vi "Tape on off.vi"(7 "Settings":T1={"max velocity"={"Value"=0.0, "Min"=0.0, "Max"=0.0, "StepSize"=0.0, "Tolerance"=0.0, "ValueActual"=0.0}, "continious velocity"={"Value"=0.0, "Min"=0.0, "Max"=0.0, "StepSize"=0.0, "Tolerance"=0.0, "ValueActual"=0.0}, "shake"=enum."off", "direction"=enum."left", "RedRatio"={"Value"=0.0, "Min"=0.0, "Max"=0.0, "StepSize"=0.0, "Tolerance"=0.0, "ValueActual"=0.0}, "StepSize"={"Value"=0.0, "Min"=0.0, "Max"=0.0, "StepSize"=0.0, "Tolerance"=0.0, "ValueActual"=0.0}, "position"={"Value"=0.0, "Min"=0.0, "Max"=0.0, "StepSize"=0.0, "Tolerance"=0.0, "ValueActual"=0.0}, "velocity"={"Value"=0.0, "Min"=0.0, "Max"=0.0, "StepSize"=0.0, "Tolerance"=0.0, "ValueActual"=0.0}, "Step"=enum."off", "Mode"=enum."on demand", "timeout"={"Value"=0.0, "Min"=0.0, "Max"=0.0, "StepSize"=0.0, "Tolerance"=0.0, "ValueActual"=0.0}, "DelayStage"={"Value"=0.0, "Min"=0.0, "Max"=0.0, "StepSize"=0.0, "Tolerance"=0.0, "ValueActual"=0.0}, "TapeMotor"=enum."off", "encoder Axis"=0, "oldpos"=0.0, "ResetEncoder"=enum."off", "tape monitor"=enum."off", "ComPort"="", "Stream Settings"={"My Name"="", "Remote IP Address"="", "Remote Name"=""}, "Motor1Axis"=0, "Motor2Axis"=0, "OptimizeTensionAfterStep"=enum."off", "StepVelocity"={"Value"=0.0, "Min"=0.0, "Max"=0.0, "StepSize"=0.0, "Tolerance"=0.0, "ValueActual"=0.0}, "MotorDirection"=enum."left", "MinTapeMonMax"={"Value"=0.0, "Min"=0.0, "Max"=0.0, "StepSize"=0.0, "Tolerance"=0.0, "ValueActual"=0.0}, "NumberSubSteps"={"Value"=0.0, "Min"=0.0, "Max"=0.0, "StepSize"=0.0, "Tolerance"=0.0, "ValueActual"=0.0}, "SimpleMinTapeMonMaxCheck"=enum."off", "WaitBeforeScanStep"={"Value"=0.0, "Min"=0.0, "Max"=0.0, "StepSize"=0.0, "Tolerance"=0.0, "ValueActual"=0.0}, "MaxStepTries"={"Value"=100.0, "Min"=0.0, "Max"=0.0, "StepSize"=0.0, "Tolerance"=0.0, "ValueActual"=0.0}}, 8 "error in (no error)":errorcluster, 9 "Arg":string, 10 "String":string, 11 "VISA Refnum in":refnum<visa-resource-name>) -> (0 "error out":errorcluster, 2 "Velocity (units/s)":dbl, 3 "new commands":string)   [LabVIEW 2020, in "TapeDrive.lvclass"]
uses:
  TapeDrive.lvclass
  settings_TypDef.ctl
  shared/numericVariable_TypeDef.ctl
  shared/OnOffTypeDef.ctl
  Direction_TypDef.ctl
  Mode_TypDEf.ctl
  <vilib>/addons/_JKI.lib/Network_Streams_Connection.llb/PublicSettings.ctl
  shared/CompressAndUpdate(Poly)/CompressAndUpdate(Enum).vi
  Newport ESP301/Newport ESP301.lvlib
  BaseDriver/BaseDriver.lvclass
  <vilib>/addons/_JKI.lib/Network_Streams_Connection.llb/NetworkConnection.lvclass
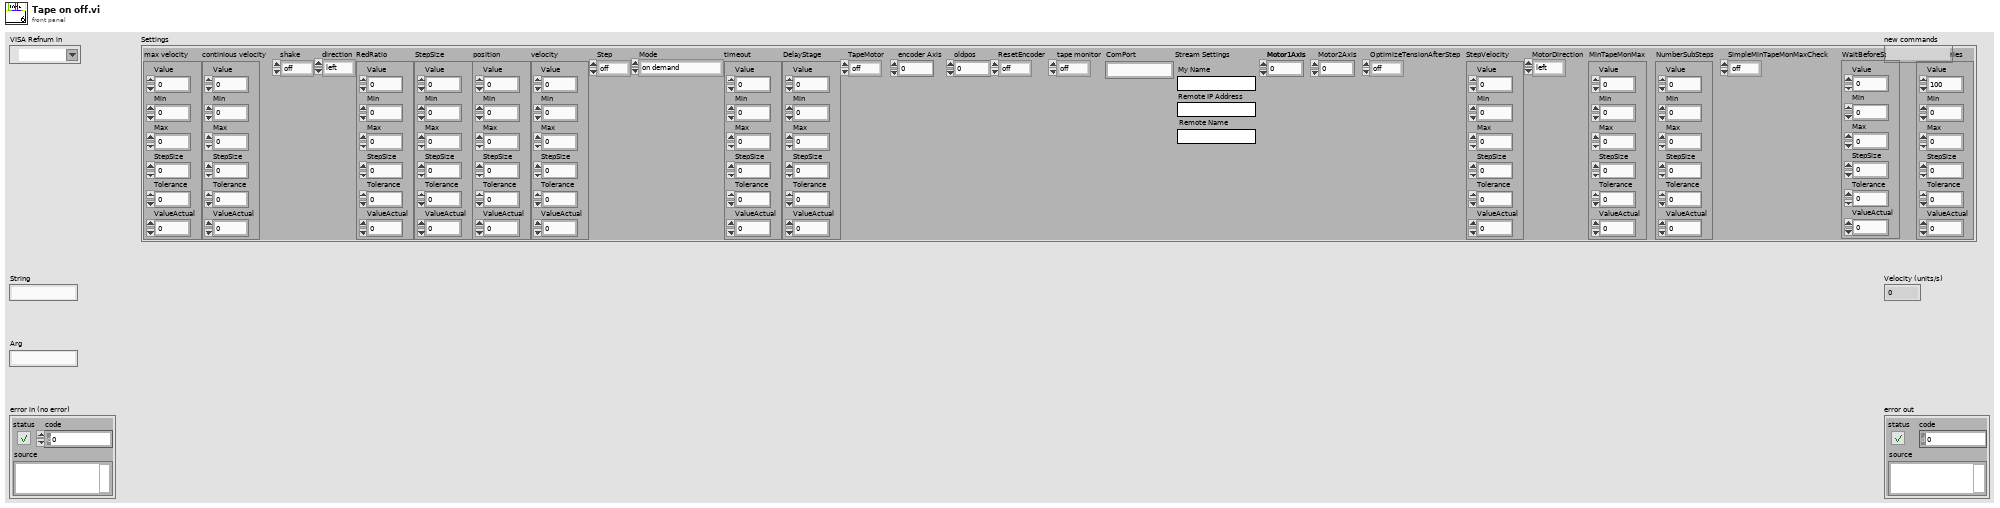
[diagram p1: front panel]
types:
  T1 = typedef "TapeDrive.lvclass/settings_TypDef.ctl" = cluster{"max velocity":T2, "continious velocity":T2, "shake":T3, "direction":T4, "RedRatio":T2, "StepSize":T2, "position":T2, "velocity":T2, "Step":T3, "Mode":T5, "timeout":T2, "DelayStage":T2, "TapeMotor":T3, "encoder Axis":i32, "oldpos":dbl, "ResetEncoder":T3, "tape monitor":T3, "ComPort":string, "Stream Settings":T6, "Motor1Axis":i32, "Motor2Axis":i32, "OptimizeTensionAfterStep":T3, "StepVelocity":T2, "MotorDirection":T4, "MinTapeMonMax":T2, "NumberSubSteps":T2, "SimpleMinTapeMonMaxCheck":T3, "WaitBeforeScanStep":T2, "MaxStepTries":T2}
  T2 = typedef "BaseDriver.lvclass/numericVariable_TypeDef.ctl" = cluster{"Value":dbl, "Min":dbl, "Max":dbl, "StepSize":dbl, "Tolerance":dbl, "ValueActual":dbl}
  T3 = typedef "OnOffTypeDef.ctl" = enum16{"off", "on"}
  T4 = typedef "Direction_TypDef.ctl" = enum16{"left", "right"}
  T5 = typedef "Mode_TypDEf.ctl" = enum16{"on demand", "continuous", "scan"}
  T6 = typedef "NetworkConnection.lvclass/PublicSettings.ctl" = cluster{"My Name":string, "Remote IP Address":string, "Remote Name":string}
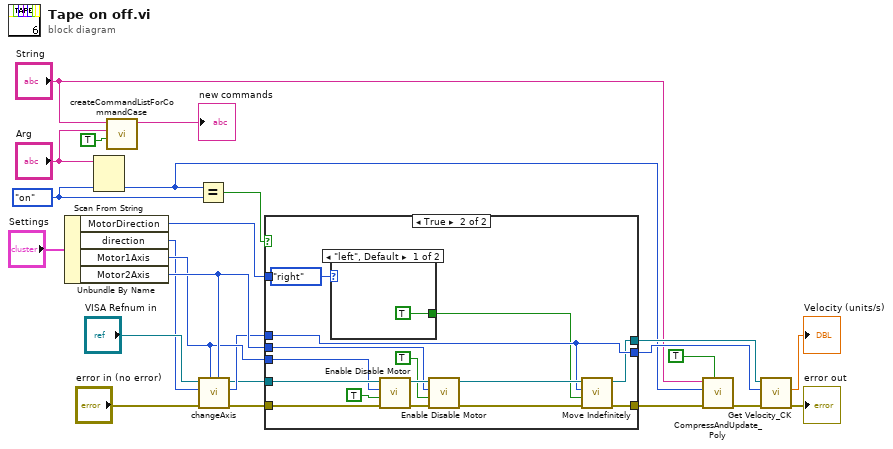
[diagram p0: block diagram]
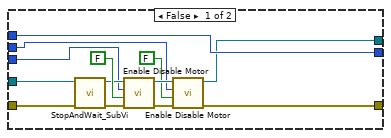
[diagram p2: hidden frame]
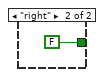
[diagram p3: hidden frame]
diagram:
  w10 = OnOffTypeDef."on" ("TapeMotor")
  n1 = Unbundle By Name("Settings") -> ("MotorDirection"=w24:T4, "direction"=w4:T4, "Motor1Axis"=w22:i32, "Motor2Axis"=w23:i32)
  n2 = Scan From String(input string="Arg", default 1=w10) -> (output 1=w13:T3)  [unwired: 3 in, 3 out]
  n3 = call "createCommandListForCommandCase.vi"("immediate Check (only once)"=TRUE, "setvalue"="Arg", "command"="String") -> ("new commands"=→"new commands":string)  [unwired: 8 in]
  n4 = Equal?(x=w13, y=w10) -> (x = y?=w11:bool)
  n5 = call "changeAxis.vi"("Motor2Axis"=w23, "Motor1Axis"=w22, "error in (no error)"="error in (no error)", "direction 2"=w4, "VISA Refnum in"="VISA Refnum in") -> ("error out"=w8:errorcluster, "Master"=w7:i32, "VISA Refnum out"=w6:refnum<visa-resource-name>)  [unwired: 3 in, 1 out]
  n6 = case shown="True" w11 {
    tunnel: w6 -> [w37 w48]
    tunnel: w7 -> [w28 w43]
    tunnel: w8 -> [w36 w46]
    tunnel: [w29 w44] -> w14
    tunnel: [w28 w43] -> w18
    tunnel: [w27 w42] -> w19
    tunnel: w22 -> [w26 w41]
    tunnel: w23 -> [w25 w40]
    tunnel: w24 -> [_ _]
    frame False {
      n7 = call "StopAndWait_SubVi.vi"("error in (no error)"=w36, "VISA Refnum in"=w37) -> ("error out"=w30:errorcluster, "VISA Refnum out"=w31:refnum<visa-resource-name>)  [unwired: 8 in]
      n8 = call "Enable Disable Motor.vi"("error in (no error)"=w30, "Action (OFF)"=FALSE, "Axis (1)"=w26, "VISA resource name"=w31) -> ("error out"=w33:errorcluster, "VISA resource name out"=w34:refnum<visa-resource-name>)  [unwired: 2 in]
      n9 = call "Enable Disable Motor.vi"("error in (no error)"=w33, "Action (OFF)"=FALSE, "Axis (1)"=w25, "VISA resource name"=w34) -> ("error out"=w29:errorcluster, "VISA resource name out"=w27:refnum<visa-resource-name>)  [unwired: 2 in]
    }
    frame True {
      n10 = case shown="\"left\", Default" Direction_TypDef."right" ("MotorDirection") {
        tunnel: [TRUE ("Move Direction (+)") FALSE ("Move Direction (+)")] -> w39
        frame "left", Default {
        }
        frame "right" {
        }
      }
      n11 = call "Enable Disable Motor.vi"("error in (no error)"=w46, "Action (OFF)"=TRUE, "Axis (1)"=w41, "VISA resource name"=w48) -> ("error out"=w50:errorcluster, "VISA resource name out"=w51:refnum<visa-resource-name>)  [unwired: 2 in]
      n12 = call "Enable Disable Motor.vi"("error in (no error)"=w50, "Action (OFF)"=TRUE, "Axis (1)"=w40, "VISA resource name"=w51) -> ("error out"=w45:errorcluster, "VISA resource name out"=w47:refnum<visa-resource-name>)  [unwired: 2 in]
      n13 = call "Move Indefinitely.vi"("error in (no error)"=w45, "Move Direction (+)"=w39, "Axis (1)"=w43, "VISA resource name"=w47) -> ("error out"=w44:errorcluster, "VISA resource name out"=w42:refnum<visa-resource-name>)  [unwired: 2 in]
    }
  }
  n14 = call-poly "CompressAndUpdate_Poly.vi"("force CVT update (false)"=TRUE, "error in"=w14, "enum variant"=w13, "command or variable name"="String") -> ("error out"=w17:errorcluster)  [unwired: 7 in]
  n15 = call "Get Velocity_CK.vi"("error in (no error)"=w17, "Axis (1)"=w18, "VISA resource name"=w19) -> ("error out"=→"error out":errorcluster, "Velocity (units/s)"=→"Velocity (units/s)":dbl)  [unwired: 2 in, 1 out]
